vi "niScope Fetch Forever.vi"() -> ()   [LabVIEW 2024]
doc: "Example: Fetch Forever\n\nRecommended Input Signal: 10 Hz, 1.8 Vpp, sine wave\n\nDevices Supported: Refer to NI Example Finder\n(You should use the 16 or 32 bit fetch functions for devices with resolutions greater than 8 bits)\n\nLabVIEW Description:\n\nThis example demonstrates using continuous acquisition to fetch an infinite record of data (or at least until you press stop). It configures and starts one acquisition that is never triggered. This is accomplished by configuring a software trigger and never sending the software trigger. Therefore, the oscilloscope will continuously acquire data into its onboard memory until Abort or Close is called. \n\nThe loop continuously fetches data from onboard memory into the computer's memory, using DMA transfers. If the sampling rate is low, the computer can fetch all the data from the oscilloscope, so data is never overwritten. However, at faster sampling rates, the computer will not be able to fetch the data before it is overwritten by new data. This results in the \"data overwritten\" error.\n\nThe input parameters to the Fetch VI include the maximum waveform size to fetch. Since a timeout of zero is set, the oscilloscope will return however many points are currently available rather than waiting for the requested number of samples. The Fetch VI will return a waveform with the actual number of points fetched. \n\nThe \"relative to\" property determines which samples to fetch from memory. In this example, it is set to the read pointer, which starts at the beginning of the acquisition and is incremented by the actual number of points during each fetch.\n\nNotice that this example uses a Binary Fetch VI. Binary fetching is faster than fetching scaled voltage data (and uses significantly less memory). The 8-bit Fetch function is suitable for any device that returns 8-bit data. However, the example should use the 16-bit Fetch for devices like the NI 5122 since this device returns higher resolution data. If you fetch 8-bit data from higher resolution devices, NI-SCOPE is actually throwing away resolution."
uses:
  <instrlib>/niScope/Acquire/Fetch/niScope Fetch Binary 8.vi
  <instrlib>/niScope/Configure/Trigger/niScope Configure Trigger Software.vi
panel:
  in  "Simulate?":bool
  in  "Stop Button":bool
  out "Last Points Fetched":i32
  out "Total Points Fetched":i32
  in  "Channel Name":string="0" caption="Channel(s)"
  in  "Plot Data?":bool=TRUE
  in  "Resource Name":refnum<k15>="Dev1" caption="Resource Name(s)"
  in  "Max. Points per Fetch":i32=1000
  out "Waveform from Scope":dbl[](graph)
  in  "Min. Sample Rate":dbl=10000000.0 format="%#_6p"
  in  "Vertical Range (V)":dbl=2.0 format="%_3g"
  # "Overview: Demonstrates using continuous acquisition to fetch an infinite record of data (or until you press stop). \nRequirements: NI-SCOPE\nInstructions: \n1.  Select the appropriate device in the Resource Name(s) control.\n2.  Enter the channels you would like to acquire from in the Channel(s) control.\n3.  Ensure the values entered in the Min Sample Rate, Vertical Range, and Max Points Per Fetch are appropriate.\n4.  Run the VI."
  # "Vertical and Horizontal"
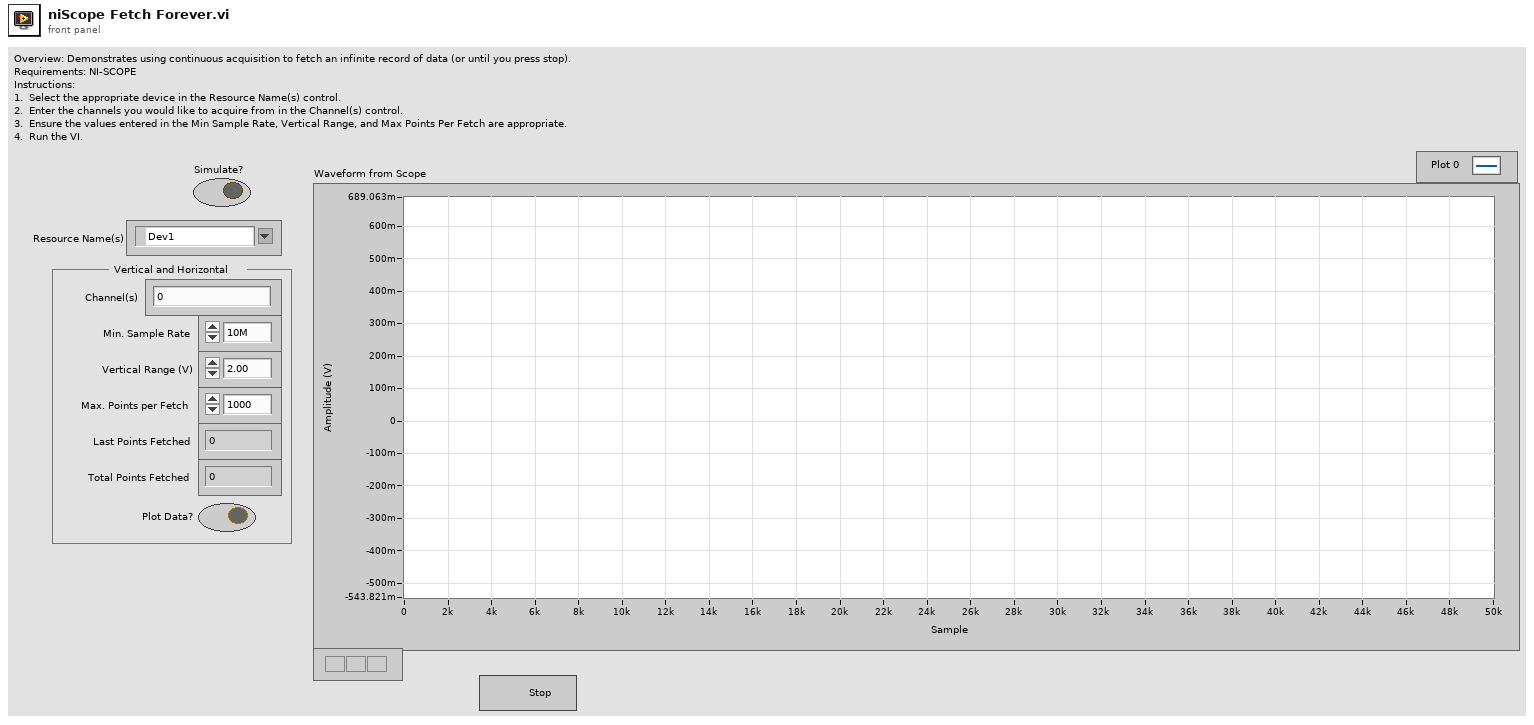
[diagram p1: front panel]
types:
  T1 = cluster{"actualSamples":i32, "absoluteInitialX":dbl, "relativeInitialX":dbl, "xIncrement":dbl, "offset":dbl, "gain":dbl, "reserved1":dbl, "reserved2":dbl}
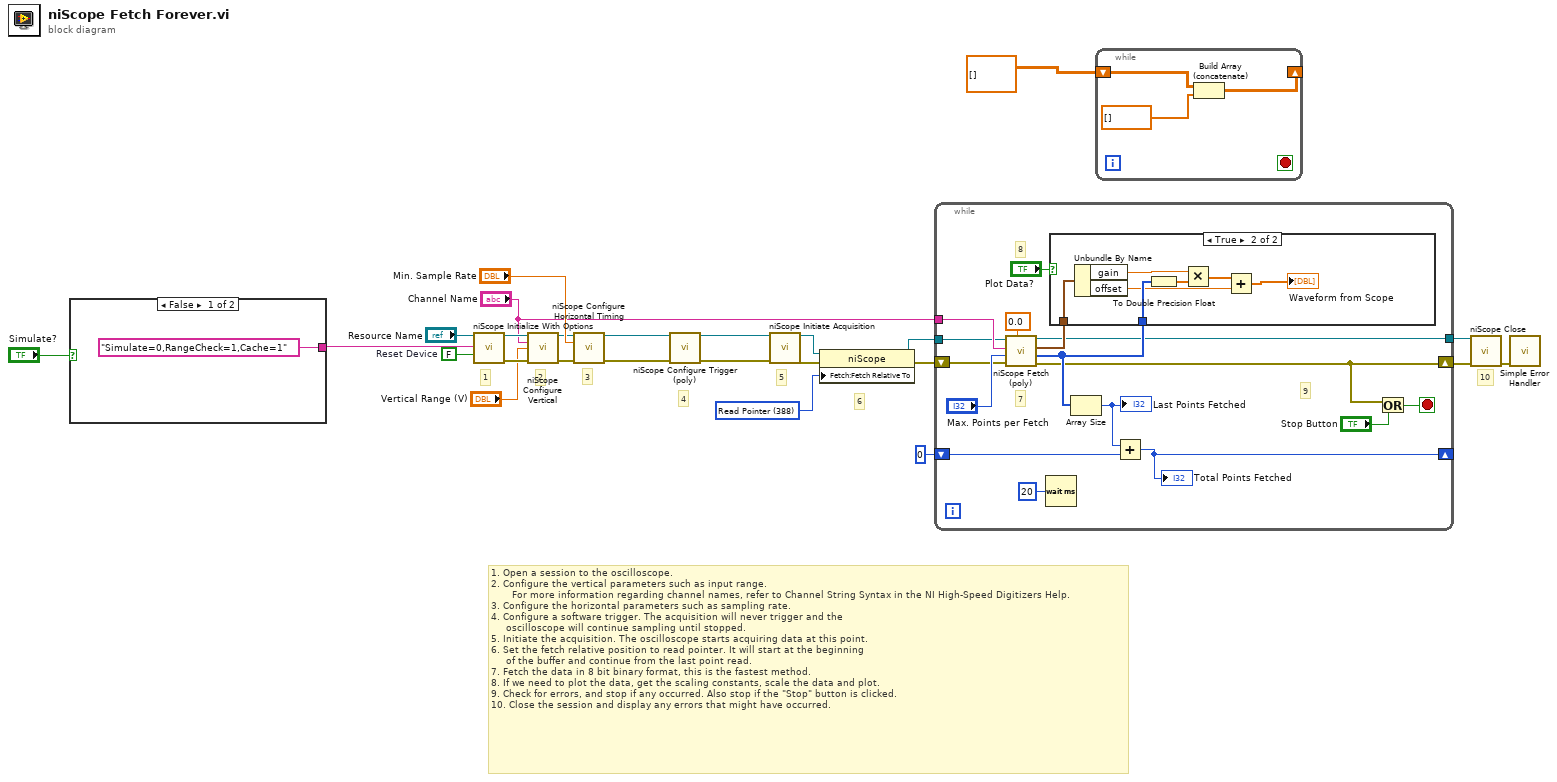
[diagram p0: block diagram]
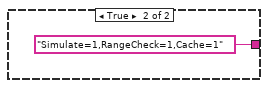
[diagram p2: hidden frame]
diagram:
  w4 = 388 items=["Start"=482, "Trigger"=483, "Pretrigger"=477, "Now"=481, "Read Pointer"=388] ("Fetch:Fetch Relative To")
  w23 = FALSE  # Reset Device
  # "1. Open a session to the oscilloscope.\n2. Configure the vertical parameters such as input range.\n       For more information regarding channel names, refer to Channel String Syntax in the NI High-Speed Digitizers Help.\n3. Configure the horizontal parameters such as sampling rate.\n4. Configure a software trigger. The acquisition will never trigger and the\n     oscilloscope will continue sampling until stopped.\n5. Initiate the acquisition. The oscilloscope starts acquiring data at this point.\n6. Set the fetch relative position to read pointer. It will start at the beginning\n     of the buffer and continue from the last point read.\n7. Fetch the data in 8 bit binary format, this is the fastest method.\n8. If we need to plot the data, get the scaling constants, scale the data and plot.\n9. Check for errors, and stop if any occurred. Also stop if the \"Stop\" button is clicked.\n10. Close the session and display any errors that might have occurred."
  # "10"
  # "6"
  # "5"
  # "4"
  # "3"
  # "2"
  # "1"
  n1 = case shown="False" "Simulate?" {
    tunnel: ["Simulate=0,RangeCheck=1,Cache=1" ("option string") "Simulate=1,RangeCheck=1,Cache=1" ("option string")] -> w2
    frame False {
    }
    frame True {
    }
  }
  n2 = call <instrlib>:"niScope Initialize With Options.vi"("resource name"="Resource Name", "option string"=w2, "reset device"=w23) -> ("instrument handle"=w25:refnum<k15>, "error out"=w24:errorcluster)  [unwired: 11 in]
  n3 = call <instrlib>:"niScope Configure Vertical.vi"("instrument handle"=w25, "channels"="Channel Name", "vertical range"="Vertical Range (V)", "error in"=w24) -> ("instrument handle out"=w15:refnum<k15>, "error out"=w14:errorcluster)  [unwired: 10 in]
  n4 = call <instrlib>:"niScope Configure Horizontal Timing.vi"("instrument handle"=w15, "min sample rate"="Min. Sample Rate", "error in"=w14) -> ("instrument handle out"=w21:refnum<k15>, "error out"=w22:errorcluster)  [unwired: 11 in]
  n5 = call-poly <instrlib>:"niScope Configure Trigger (poly).vi"("instrument handle"=w21, "error in"=w22) -> ("instrument handle out"=w17:refnum<k15>, "error out"=w16:errorcluster)  [unwired: 12 in]
  n6 = call <instrlib>:"niScope Initiate Acquisition.vi"("instrument handle"=w17, "error in"=w16) -> ("instrument handle out"=w9:refnum<k15>, "error out"=w12:errorcluster)  [unwired: 12 in]
  n7 = property class="niScope"(reference=w9, error in=w12, "Fetch:Fetch Relative To"=w4) -> (reference out=w8:refnum<k15>, error out=w7:errorcluster)
  n8 = while {
    shift-left: 0 -> [w43]
    shift-right: [w40] -> _
    tunnel: "Channel Name" -> [w41]
    tunnel: w8 -> [w32]
    tunnel: [w30] -> w5
    shift-right: [w28] -> w6
    shift-left: w7 -> [w31]
    stop <- w42 stop-if-true
    # "9"
    # "8"
    # "7"
    n9 = call-poly <instrlib>:"niScope Fetch (poly).vi"("timeout"=0.0, "error in"=w31, "numSamples"="Max. Points per Fetch", "channels"=w41, "instrument handle"=w32) -> ("error out"=w28:errorcluster, "wfm"=w37:i8[], "wfm info"=w35:T1, "instrument handle out"=w30:refnum<k15>)  [unwired: 3 in]
    n10 = Wait (ms)(milliseconds to wait=u32 20) -> ()  [unwired: 1 out]
    n11 = case shown="True" "Plot Data?" {
      tunnel: w37 -> [_ w49]
      tunnel: w35 -> [_ w50]
      frame False {
      }
      frame True {
        n12 = Unbundle By Name(w50) -> ("gain"=w48:dbl, "offset"=w46:dbl)
        n13 = To Double Precision Float(number=w49) -> (double precision float=w44:dbl[])
        n14 = Multiply(x=w48, y=w44) -> (x*y=w47:dbl[])
        n15 = Add(x=w47, y=w46) -> (x+y=→"Waveform from Scope":dbl[])
      }
    }
    n16 = Array Size(array=w37) -> (size(s)=w36:i32)
    "Last Points Fetched" <- w36
    n17 = Add(x=w36, y=w43) -> (x+y=w40:i32)
    "Total Points Fetched" <- w40
    n18 = Or(x=w28, y="Stop Button") -> (x .or. y?=w42:bool)
  }
  n19 = while {
    shift-right: [w52] -> _
    shift-left: dbl[][] [] -> [w51]
    stop <- _ stop-if-true
    n20 = Build Array (concatenate)(w51, dbl[] []) -> (w52:dbl[][])
  }
  n21 = call <instrlib>:"niScope Close.vi"("instrument handle"=w5, "error in"=w6) -> ("error out"=w11:errorcluster)  [unwired: 13 in]
  n22 = call <vilib>:"Simple Error Handler.vi"("error in (no error)"=w11) -> ()  [unwired: 4 in, 5 out]
